vi "Phasor Compare Frequencies.vi"(8 "Phasor Frequency 2 Name":string="Phasor Frequency 2", 9 "Phasor Frequency 2":dbl[unit], 10 "Phasor Frequency 1 Name":string="Phasor Frequency 1", 11 "Phasor Frequency 1":dbl[unit]) -> (3 "Accept?":bool)   [LabVIEW 2021, in "Phasor.lvlib"]
uses:
  c9340793-c582-4770-84bb-cfb0e3ea166d.vi
  c9340793-c582-4770-84bb-cfb0e3ea166d.vi/8a80743f-1319-44c8-96b0-3ef8fc688731.vi
  c9340793-c582-4770-84bb-cfb0e3ea166d.vi/931f4f8f-d8c6-4056-833f-5c8fe97b24b9.vi
  Phasor.lvlib
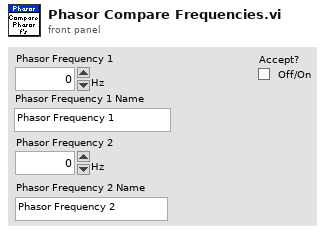
[diagram p1: front panel]
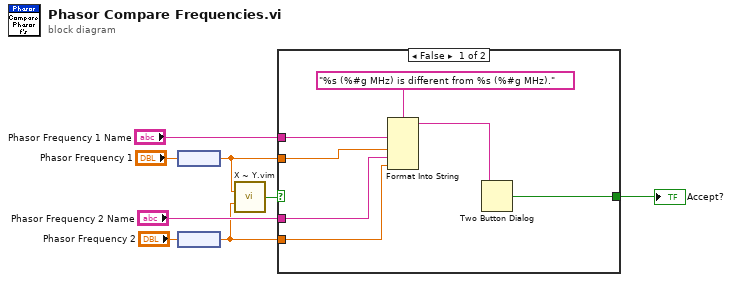
[diagram p0: block diagram]
diagram:
  n1 = node("Phasor Frequency 1") -> (w2:dbl)
  n2 = node("Phasor Frequency 2") -> (w1:dbl)
  n3 = call "X ~ Y.vim"("X"=w2, "Y"=w1) -> ("X ~= Y?"=w8:bool)  [unwired: 13 in]
  n4 = case shown="False" w8 {
    selector: w8 -> [_ w16]
    tunnel: [w11 w16] -> w7
    tunnel: "Phasor Frequency 1 Name" -> [w13 _]
    tunnel: "Phasor Frequency 2 Name" -> [w12 _]
    tunnel: w2 -> [w10 _]
    tunnel: w1 -> [w9 _]
    frame False {
      n5 = Format Into String(format string="%s (%#g MHz) is different from %s (%#g MHz).", w13, w10, w12, w9) -> (resulting string=w14:string)  [unwired: 2 in, 1 out]
      n6 = Two Button Dialog(message=w14) -> (T button?=w11:bool)  [unwired: 2 in]
    }
    frame True {
    }
  }
  "Accept?" <- w7
